vi "Set Default.vi"(8 "error in (no error)":errorcluster, 11 "DMM Immediate Measure Msg in":refnum<class "DMM Immediate Measure Msg.lvclass">) -> (0 "error out":errorcluster, 3 "DMM Immediate Measure Msg out":refnum<class "DMM Immediate Measure Msg.lvclass">)   [LabVIEW 2020, in "DMM Msg.lvlib" / "DMM Immediate Measure Msg.lvclass"]
doc: "Restore private data to a defined default state.\n\nThis implementation sets:\n1 measurement with -1 Max Time\nRestore Range TRUE\nAwait reply, -1ms timeout at normal priority with publish"
uses:
  DMM Immediate Measure Msg.lvclass
  PPL/HDH.Actor Framework.Core.Actor.lvlibp/1abvi3w/vi.lib/ActorFramework/Message Enqueuer/Message Priority.ctl
  PPL/HDH.Actor Framework.Core.Publisher.lvlibp/Messages/Response Msg/Response Core/Controls/Ctl_SendFunction.ctl
  DMM Immediate Measure Msg.lvclass/DMM Immediate Measure Msg.ctl
  DMM Msg/DMM Msg.lvclass
  PPL/HDH.Actor Framework.Core.Instrument Handler.lvlibp/Messages/Instrument Msg/Instrument Msg.lvclass
  PPL/HDH.Actor Framework.Core.Publisher.lvlibp
  PPL/HDH.Actor Framework.Core.Actor.lvlibp/1abvi3w/vi.lib/ActorFramework/Message Enqueuer/Message Enqueuer.lvclass
  C:/Current projects/WS/PPL/HDH.Actor Framework.Core.Instrument Handler.lvlibp/Messages/Instrument Msg/Instrument Msg.lvclass
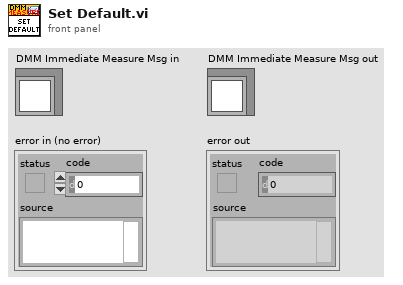
[diagram p1: front panel]
types:
  T1 = typedef "HDH.Actor Framework.Core.Publisher.lvlibp/Ctl_SendFunction.ctl" = enum16{"Send and Forget", "Request Reply", "Await Reply"}
  T2 = typedef "HDH.Actor Framework.Core.Actor.lvlibp/Message Enqueuer.lvclass/Message Priority.ctl" = enum16{"Low", "Normal", "High"}
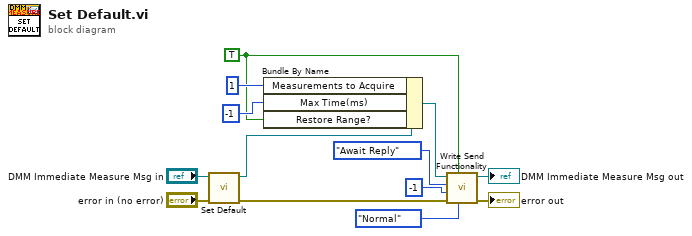
[diagram p0: block diagram]
diagram:
  w1 = TRUE ("Publish Data?(T)")
  n1 = call-parent "Set Default.vi"("error in (no error)"="error in (no error)", "Flex Msg in"="DMM Immediate Measure Msg in") -> ("error out"=w8:errorcluster, "Flex Msg out"=w13:refnum<class "DMM Immediate Measure Msg.lvclass">)  [unwired: 8 in]
  n2 = Bundle By Name(cluster=w13, "Measurements to Acquire"=1, "Max Time(ms)"=-1, "Restore Range?"=w1) -> (w10:refnum<class "DMM Immediate Measure Msg.lvclass">)
  n3 = call "Write Send Functionality.vi"("Message Priority(Normal)"=Message_Priority."Normal", "Publish Data?(T)"=w1, "error in (no error)"=w8, "Timeout if Waiting(-1ms)"=-1, "Send Function(Await Reply)"=Ctl_SendFunction."Await Reply", "Instrument Msg in"=w10) -> ("error out"=→"error out":errorcluster, "Instrument Msg out"=→"DMM Immediate Measure Msg out":refnum<class "DMM Immediate Measure Msg.lvclass">)  [unwired: 4 in]
